vi "MICSD Serial Read.vi"(7 "Timeout(mS)":dbl=3000.0, 8 "error in (no error)":errorcluster, 11 "VISA Resource Name":refnum<visa-resource-name>) -> (0 "error out":errorcluster, 2 "Read Data":u8[](array[numeric]) format="%02x", 3 "DUP Visa Resource Name":refnum<visa-resource-name>)   [LabVIEW 2020]
panel:
  in  "Block Ctl(F)":bool=TRUE
  in  "Logger (Debug)":bool
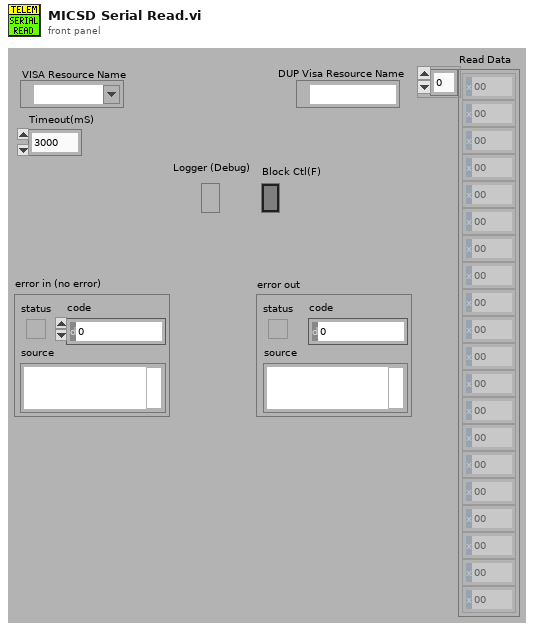
[diagram p1: front panel]
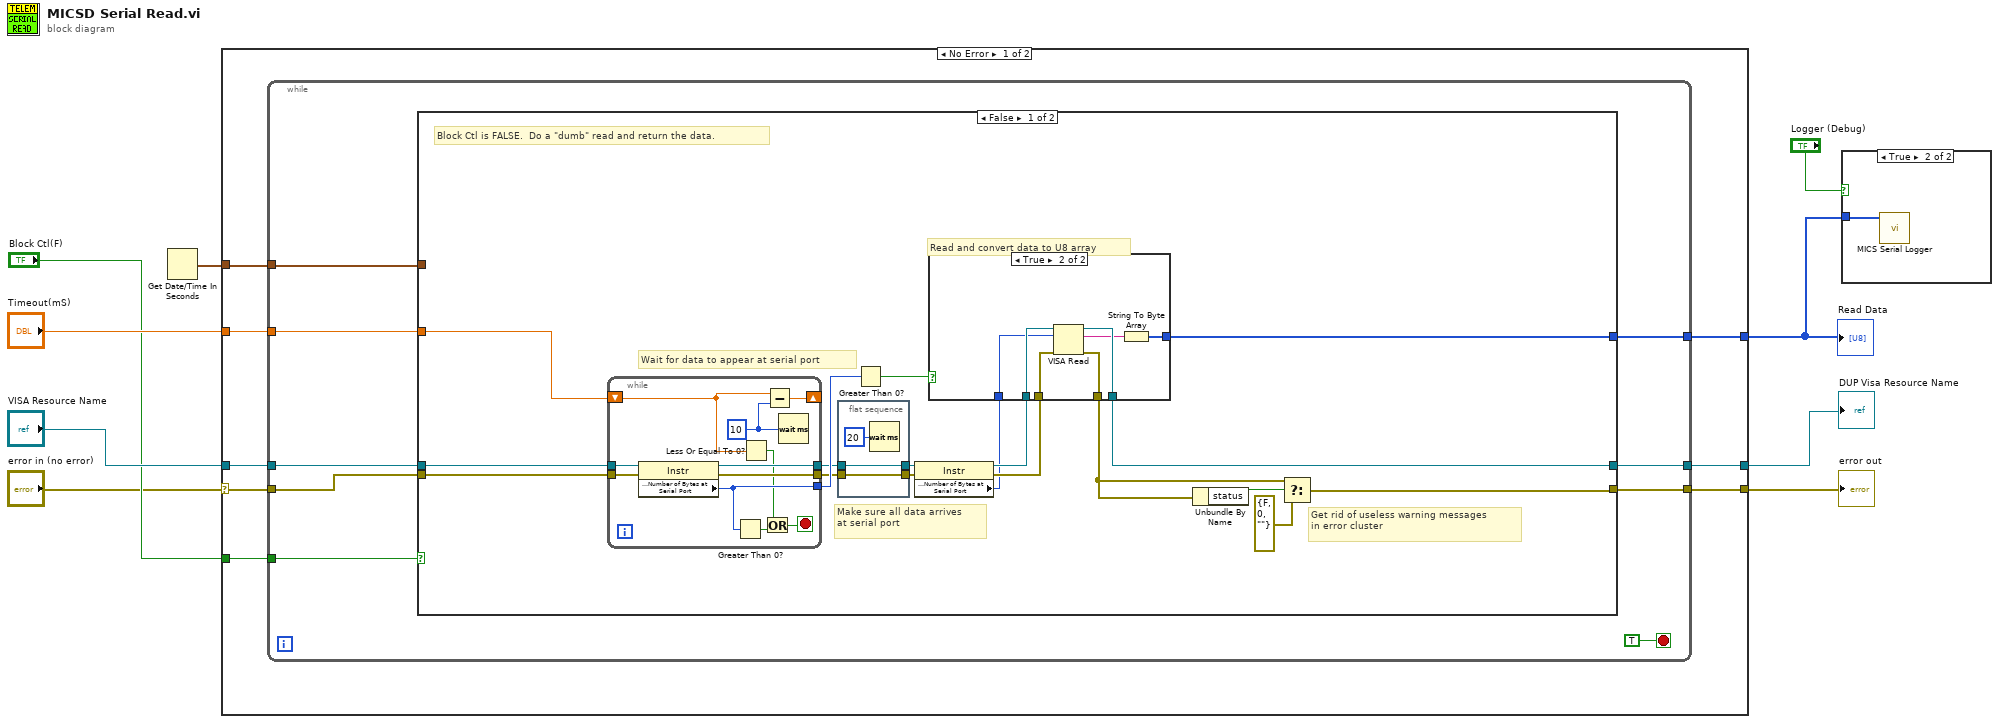
[diagram p0: block diagram]
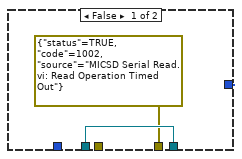
[diagram p2: hidden frame]
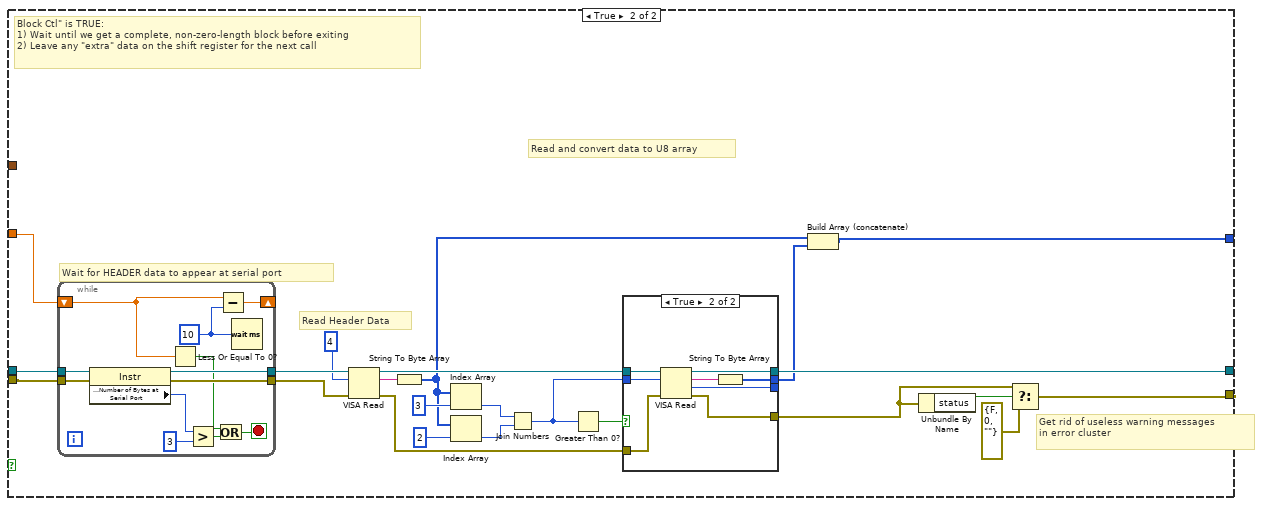
[diagram p3: hidden frame]
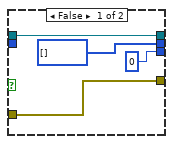
[diagram p4: hidden frame]
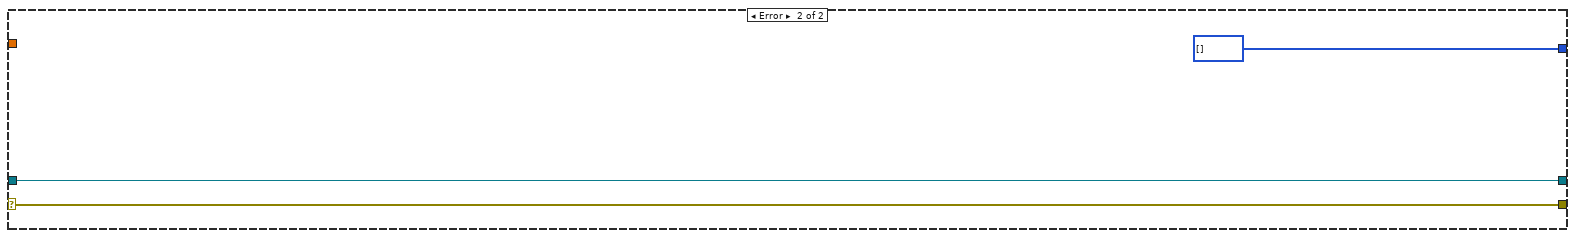
[diagram p5: hidden frame]
diagram:
  n1 = Get Date/Time In Seconds() -> (seconds since 1Jan1904=w1:timestamp)
  n2 = case shown="No Error" "error in (no error)" {
    selector: "error in (no error)" -> [w11 w116]
    tunnel: "VISA Resource Name" -> [w17 w117]
    tunnel: [w16 w117] -> w8
    tunnel: [w15 w116] -> w7
    tunnel: "Timeout(mS)" -> [w14 _]
    tunnel: [w13 u8[] [] ("unsigned byte array")] -> w5
    tunnel: "Block Ctl(F)" -> [w12 _]
    tunnel: w1 -> [w10 _]
    frame No Error {
      n3 = while {
        tunnel: w17 -> [w26]
        tunnel: w11 -> [w25]
        tunnel: [w24] -> w16
        tunnel: [w23] -> w15
        tunnel: w14 -> [w22]
        tunnel: [w21] -> w13
        tunnel: w12 -> [w20]
        tunnel: w10 -> [w19]
        stop <- TRUE stop-if-true
        n4 = case shown="False" w20 {
          tunnel: w26 -> [w44 w87]
          tunnel: w25 -> [w43 w86]
          tunnel: [w42 w81] -> w24
          tunnel: [w41 w89] -> w23
          tunnel: w22 -> [w40 w88]
          tunnel: [w27 w69] -> w21
          tunnel: w19 -> [_ _]
          frame False {
            # "Block Ctl is FALSE.  Do a \"dumb\" read and return the data."
            # "Make sure all data arrives\nat serial port"
            # "Read and convert data to U8 array"
            # "Wait for data to appear at serial port"
            # "Get rid of useless warning messages\nin error cluster"
            n5 = while {
              tunnel: [w58] -> w29
              tunnel: [w57] -> w31
              tunnel: w44 -> [w56]
              tunnel: w43 -> [w55]
              tunnel: [w53] -> w38
              shift-right: [w54] -> _
              shift-left: w40 -> [w49]
              stop <- w51 stop-if-true
              w50 = u32 10 ("milliseconds to wait")
              n6 = property class="Instr"(reference=w56, error in=w55) -> (reference out=w58:refnum<visa-resource-name>, error out=w57:errorcluster, "Serial Settings:Number of Bytes at Serial Port"=w53:u32)
              n7 = Greater Than 0?(x=w53) -> (x > 0?=w52:bool)
              n8 = Less Or Equal To 0?(x=w49) -> (x <= 0?=w48:bool)
              n9 = Or(x=w48, y=w52) -> (x .or. y?=w51:bool)
              n10 = Subtract(x=w49, y=w50) -> (x-y=w54:dbl)
              n11 = Wait (ms)(milliseconds to wait=w50) -> ()  [unwired: 1 out]
            }
            n12 = flat-sequence {
              tunnel: w31 -> [w47]
              tunnel: [w47] -> w30
              tunnel: w29 -> [w45]
              tunnel: [w45] -> w28
              frame #0 {
                n13 = Wait (ms)(milliseconds to wait=u32 20) -> ()  [unwired: 1 out]
              }
            }
            n14 = Greater Than 0?(x=w38) -> (x > 0?=w39:bool)
            n15 = property class="Instr"(reference=w28, error in=w30) -> (reference out=w37:refnum<visa-resource-name>, error out=w36:errorcluster, "Serial Settings:Number of Bytes at Serial Port"=w35:u32)
            n16 = case shown="True" w39 {
              tunnel: w36 -> [_ w68]
              tunnel: w37 -> [w61 w67]
              tunnel: [errorcluster {"status"=TRUE, "code"=1002, "source"="MICSD Serial Read.vi: Read Operation Timed Out"} ("error out") w66] -> w34
              tunnel: [w61 w65] -> w42
              tunnel: [u8[] [] w62] -> w27
              tunnel: w35 -> [_ w64]
              frame False {
              }
              frame True {
                n17 = VISA Read(VISA resource name=w67, byte count=w64, error in (no error)=w68) -> (VISA resource name out=w65:refnum<visa-resource-name>, read buffer=w63:string, error out=w66:errorcluster)  [unwired: 1 out]
                n18 = String To Byte Array(string=w63) -> (unsigned byte array=w62:u8[])
              }
            }
            n19 = Unbundle By Name(w34) -> ("status"=w33:bool)
            n20 = Select(t=w34, s=w33, f=errorcluster {"status"=FALSE, "code"=0, "source"=""} ("error out")) -> (s? t:f=w41:errorcluster)
          }
          frame True {
            # "Read Header Data"
            # "Read and convert data to U8 array"
            # "Wait for HEADER data to appear at serial port"
            # "Get rid of useless warning messages\nin error cluster"
            # "Block Ctl\" is TRUE:\n1) Wait until we get a complete, non-zero-length block before exiting\n2) Leave any \"extra\" data on the shift register for the next call"
            n21 = while {
              tunnel: [w103] -> w85
              tunnel: [w102] -> w83
              tunnel: w87 -> [w101]
              tunnel: w86 -> [w100]
              shift-right: [w99] -> _
              shift-left: w88 -> [w95]
              stop <- w97 stop-if-true
              w96 = u32 10 ("milliseconds to wait")
              n22 = property class="Instr"(reference=w101, error in=w100) -> (reference out=w103:refnum<visa-resource-name>, error out=w102:errorcluster, "Serial Settings:Number of Bytes at Serial Port"=w93:u32)
              n23 = Less Or Equal To 0?(x=w95) -> (x <= 0?=w94:bool)
              n24 = Greater?(x=w93, y=u32 3) -> (0:w98:bool)
              n25 = Or(x=w94, y=w98) -> (x .or. y?=w97:bool)
              n26 = Subtract(x=w95, y=w96) -> (x-y=w99:dbl)
              n27 = Wait (ms)(milliseconds to wait=w96) -> ()  [unwired: 1 out]
            }
            n28 = VISA Read(VISA resource name=w85, byte count=u32 4, error in (no error)=w83) -> (VISA resource name out=w82:refnum<visa-resource-name>, read buffer=w78:string, error out=w77:errorcluster)  [unwired: 1 out]
            n29 = String To Byte Array(string=w78) -> (unsigned byte array=w71:u8[])
            n30 = Index Array(array=w71, index=3) -> (element=w74:u8)
            n31 = Index Array(array=w71, index=2) -> (element=w73:u8)
            n32 = Join Numbers(hi=w74, lo=w73) -> ((hi.lo)=w72:u16)
            n33 = Greater Than 0?(x=w72) -> (x > 0?=w91:bool)
            n34 = case shown="True" w91 {
              tunnel: w82 -> [w105 w115]
              tunnel: [w104 w114] -> w80
              tunnel: [w105 w113] -> w81
              tunnel: [u8[] [] w111] -> w70
              tunnel: [u32 0 ("return count") w110] -> _
              tunnel: w72 -> [_ w109]
              tunnel: w77 -> [w104 w108]
              frame False {
              }
              frame True {
                n35 = VISA Read(VISA resource name=w115, byte count=w109, error in (no error)=w108) -> (VISA resource name out=w113:refnum<visa-resource-name>, read buffer=w112:string, return count=w110:u32, error out=w114:errorcluster)
                n36 = String To Byte Array(string=w112) -> (unsigned byte array=w111:u8[])
              }
            }
            n37 = Build Array (concatenate)(w71, w70) -> (w69:u8[])
            n38 = Unbundle By Name(w80) -> ("status"=w79:bool)
            n39 = Select(t=w80, s=w79, f=errorcluster {"status"=FALSE, "code"=0, "source"=""} ("error out")) -> (s? t:f=w89:errorcluster)
          }
        }
      }
    }
    frame Error {
    }
  }
  "DUP Visa Resource Name" <- w8
  "error out" <- w7
  "Read Data" <- w5
  n40 = case shown="True" "Logger (Debug)" {
    tunnel: w5 -> [_ w119]
    frame False {
    }
    frame True {
      n41 = call "MICS Serial Logger.vi"("Array"=w119) -> ()  [unwired: 11 in]
    }
  }
